vi "Write PLL Mode.vi"(10 "PLL Mode":T1, 11 "Spectrum Analyzer in":refnum<class "Spectrum Analyzer.lvclass">) -> (3 "Spectrum Analyzer out":refnum<class "Spectrum Analyzer.lvclass">)   [LabVIEW 2020, in "Spectrum Analyzer.lvclass"]
uses:
  Spectrum Analyzer.lvclass
  Controls/PLL Mode.ctl
  Spectrum Analyzer.lvclass/Spectrum Analyzer.ctl
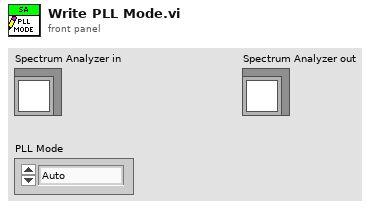
[diagram p1: front panel]
types:
  T1 = typedef "Spectrum Analyzer.lvclass/PLL Mode.ctl" = enum16{"Auto", "Narrow", "Normal", "Wide"}
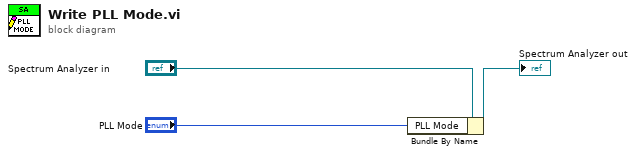
[diagram p0: block diagram]
diagram:
  n1 = Bundle By Name(cluster="Spectrum Analyzer in", "PLL Mode"="PLL Mode") -> (→"Spectrum Analyzer out":refnum<class "Spectrum Analyzer.lvclass">)
